vi "Sync - Get All Instrument Names.vi"(0 "TSM context":T1, 11 "error in":errorcluster) -> (4 "TSM context out":T1, 6 "Instrument Names":string[](array[string]), 8 "Channel Lists":string[](array[string]), 10 "Channel Group Ids":string[](array[string]), 15 "error out":errorcluster)   [LabVIEW 2020]
doc: "Returns Instrument Names for all NI-Sync instruments in the Semiconductor Module Context. You can use Instrument Names to open driver sessions."
uses:
  <vilib>/NI_TestStand_SemiconductorModule/NI_TestStand_Semiconductor_Module.lvlibp/PinMap/General/SemiconductorModuleContext.ctl
  <vilib>/NI_TestStand_SemiconductorModule/NI_TestStand_Semiconductor_Module.lvlibp
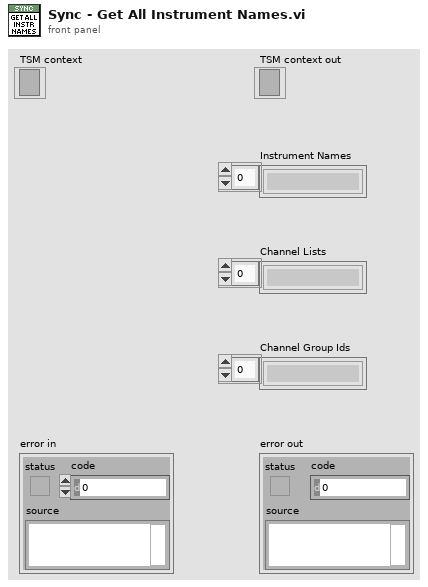
[diagram p1: front panel]
types:
  T1 = typedef "NI_TestStand_Semiconductor_Module.lvlibp/SemiconductorModuleContext.ctl" = refnum<k7>
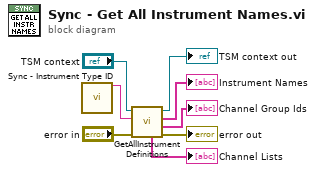
[diagram p0: block diagram]
diagram:
  n1 = call "Sync - Instrument Type ID.vi"() -> ("Instrument Type ID"=w1:string)  [unwired: 15 in]
  n2 = call <vilib>:"GetAllInstrumentDefinitions.vi"("error in (no error)"="error in", "Instrument Type Id"=w1, "Semiconductor Module Context"="TSM context") -> ("error out"=→"error out":errorcluster, "Channel Group Ids"=→"Channel Group Ids":string[], "Instrument Names"=→"Instrument Names":string[], "Semiconductor Module Context Out"=→"TSM context out":T1, "Channel Lists"=→"Channel Lists":string[])  [unwired: 4 in]
